vi "Main.vi"(11 "Module Admin":refnum<class "Delacor_lib_QMH_Module Admin.lvclass">) -> ()   [LabVIEW 2019, in "Spectrometer.lvlib"]
doc: "This template is based off of the Queued Message Handler design pattern and the Queued Message Handler project template that ships with LabVIEW.\n\nThe main difference is that the queue is private to this module and communication between modules is performed via Broadcast and Request events.\n\nRequest events are wrapped in public API methods and are handled in the Event Handling Loop (EHL) of this VI. Any module can register for Broadcast events sent by this module. The EHL generates messages based on user interface actions.\n\nThe Message Handling Loop (MHL) processes messages generated by the EHL, or by other messages. The messages are string values, so new messages can be added easily to the Message Cases case structure in the MHL. Each message cluster can also provide an optional value for Message Data, which is a variant that can be converted to whatever message-specific data is required.\n_____\nBased on Delacor QMH Project Template 5.0.0.82."
uses:
  Spectrometer.lvlib
  <vilib>/Delacor/Delacor QMH/Libraries/Module Admin_class/Delacor_lib_QMH_Module Admin.lvclass
  Module Data--cluster.ctl
  Spectrometer-LVClass/Abstract Spectrometer_class/Abstract Spectrometer.lvclass
  <vilib>/Delacor/Delacor QMH/Libraries/Message Queue_class/Delacor_lib_QMH_Message Queue.lvclass/Delacor_lib_QMH_Message Queue.ctl
  Stop Argument--cluster.ctl
  <vilib>/Delacor/Delacor QMH/Libraries/Module Admin_class/Delacor_lib_QMH_Module Admin.lvclass/Delacor_lib_QMH_Module Admin.ctl
  Set Wavelength Argument--cluster.ctl
  Set Wavelength (Reply Payload)--cluster.ctl
  Set Slit Width Argument--cluster.ctl
  Set Slit Width (Reply Payload)--cluster.ctl
  Set Grating Argument--cluster.ctl
  Set Grating (Reply Payload)--cluster.ctl
  Get Module Data Argument--cluster.ctl
  Get Module Data (Reply Payload)--cluster.ctl
  <vilib>/Utility/miscctls.llb/LVPointTypeDef.ctl
  Spectrometer-LVClass/Simulated_class/Simulated.lvclass
  C:/Users/Michael/Documents/GitHub/CampenLab/Spectrometer-LVClass/Abstract Spectrometer_class/Abstract Spectrometer.lvclass
  <vilib>/Delacor/Delacor QMH/Libraries/Message Queue_class/Delacor_lib_QMH_Enqueue Message (Single).vi
  <vilib>/Delacor/Delacor QMH/Libraries/Module Admin_class/Delacor_lib_QMH_Get External Launch.vi
  <vilib>/Utility/error.llb/Error Cluster From Error Code.vi
  <vilib>/ErrorRing/Error Ring.xnode
  <vilib>/Delacor/Delacor QMH/Libraries/Message Queue_class/Delacor_lib_QMH_Message Queue.lvclass
panel:
  in  "Spectrometer Class":u16(ring) items=["Simulated", "SpectraPro HRS"]
  out "Status":string
  in  "Simulate MHL Error":bool
  in  "Simulate EHL Error":bool
  out "error out":errorcluster
  # "SpectraPro"
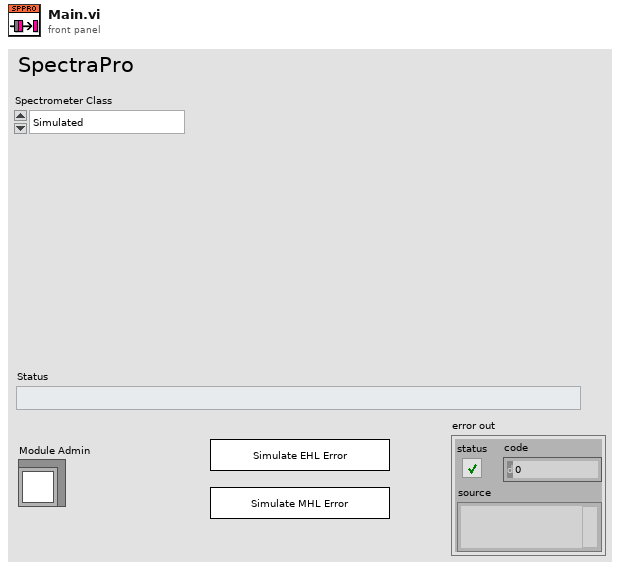
[diagram p1: front panel]
types:
  T1 = typedef "Spectrometer.lvlib/Request Events--cluster.ctl" = cluster{"Stop Module":refnum<user-event>, "Show Panel":refnum<user-event>, "Hide Panel":refnum<user-event>, "Get Module Execution Status":refnum<user-event>, "Show Diagram":refnum<user-event>, "Set Wavelength":refnum<user-event>, "Set Slit Width":refnum<user-event>, "Set Grating":refnum<user-event>, "Get Module Data":refnum<user-event>}
  T2 = typedef "Spectrometer.lvlib/Module Data--cluster.ctl" = cluster{"Status":string, "-Abstract Spectrometer.lvclass":refnum<class "Abstract Spectrometer.lvclass">, "Device Data":cluster{"Wavelength":dbl, "Slit Width":dbl, "Grating ID":u32}}
  T3 = enum32{"invalid lock state", "Not Locked", "Locked (No Password)", "Password-protected"}
  T4 = typedef "Spectrometer.lvlib/Stop Argument--cluster.ctl" = cluster{"Origin":string, "Exit via Stop Module Req?":bool, "Wait for Module to stop?":bool}
  T5 = typedef "Spectrometer.lvlib/Set Wavelength Argument--cluster.ctl" = cluster{"Wavelength":dbl, "Wait Notifier":refnum<notifier>, "wait for reply":bool}
  T6 = typedef "Spectrometer.lvlib/Set Slit Width Argument--cluster.ctl" = cluster{"Slit Width (um)":dbl, "Wait Notifier":refnum<notifier>, "wait for reply":bool}
  T7 = typedef "Spectrometer.lvlib/Set Grating Argument--cluster.ctl" = cluster{"Grating ID":u32, "Wait Notifier":refnum<notifier>, "wait for reply":bool}
  T8 = typedef "Spectrometer.lvlib/Get Module Data Argument--cluster.ctl" = cluster{"Wait Notifier":refnum<notifier>, "wait for reply":bool}
  T9 = typedef "LVPointTypeDef.ctl" = cluster{"Horizontal":i16, "Vertical":i16}
  T10 = enum32{"Invalid", "Standard", "Closed", "Hidden", "Minimized", "Maximized"}
  T11 = typedef "Spectrometer.lvlib/Set Wavelength (Reply Payload)--cluster.ctl" = cluster{"Wavelength":dbl, "Set Wavelength_error":errorcluster}
  T12 = typedef "Spectrometer.lvlib/Set Slit Width (Reply Payload)--cluster.ctl" = cluster{"Slit Width (um)":dbl, "Set Slit Width_error":errorcluster}
  T13 = typedef "Spectrometer.lvlib/Set Grating (Reply Payload)--cluster.ctl" = cluster{"Grating ID":u32, "Set Grating_error":errorcluster}
  T14 = typedef "Spectrometer.lvlib/Get Module Data (Reply Payload)--cluster.ctl" = cluster{"Spectrometer":T2, "Get Module Data_error":errorcluster}
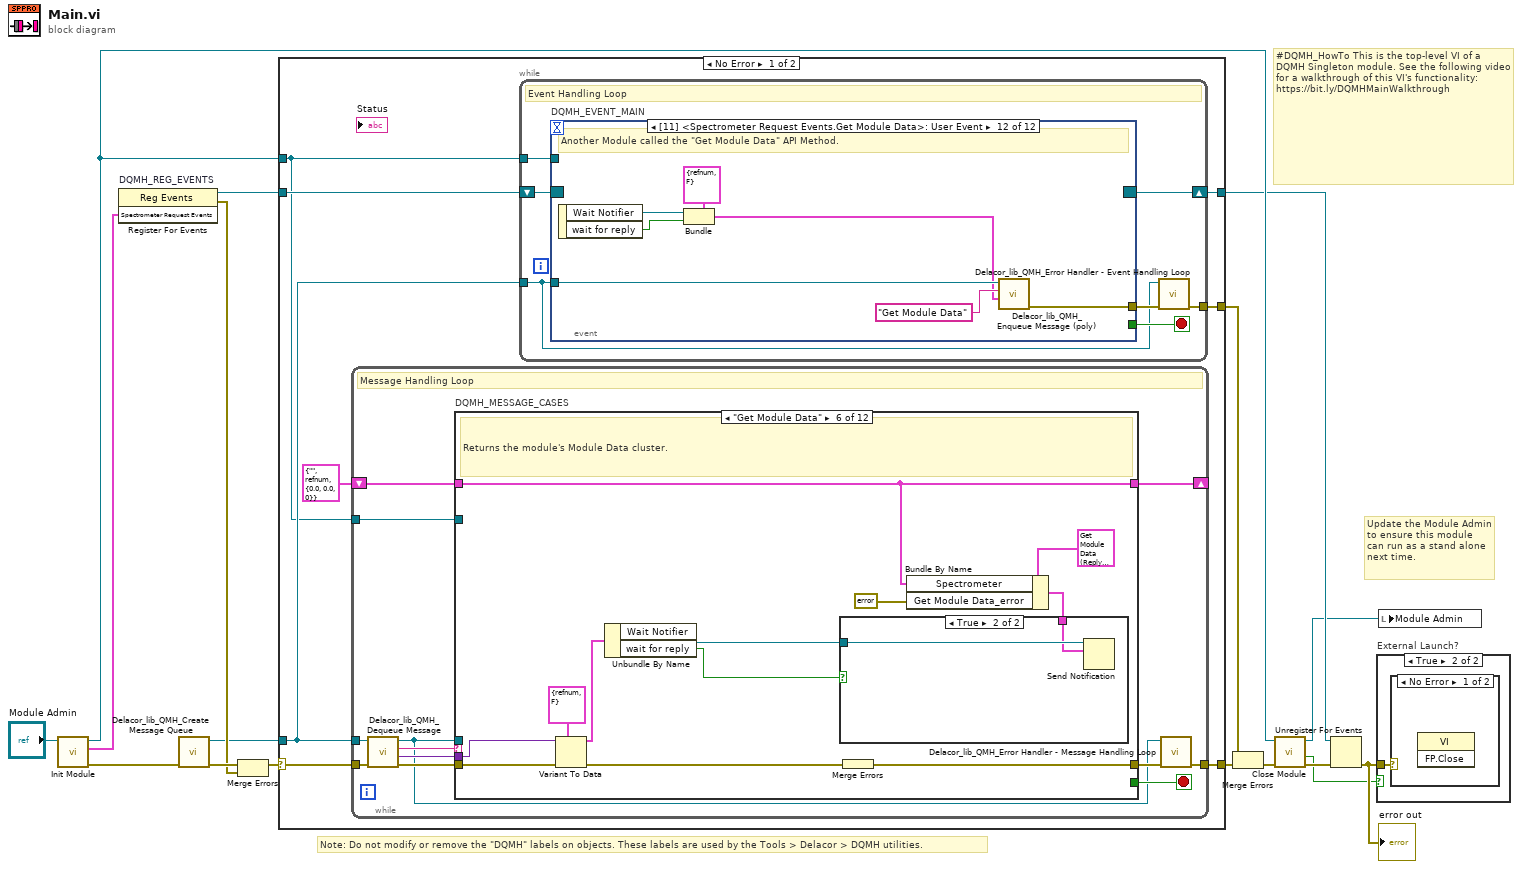
[diagram p0: block diagram]
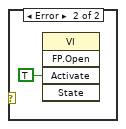
[diagram p3: hidden frame]
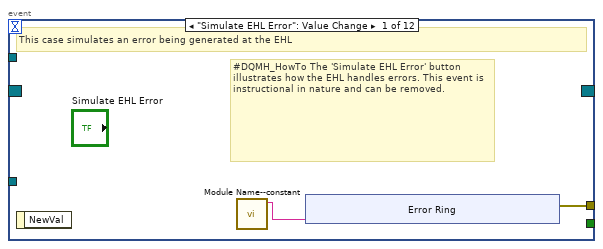
[diagram p4: hidden frame]
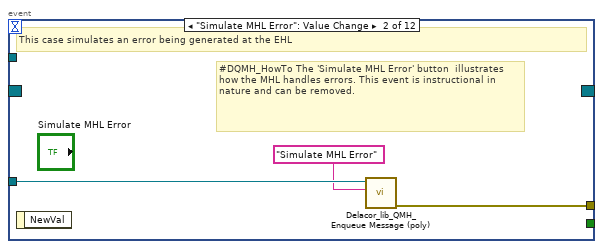
[diagram p5: hidden frame]
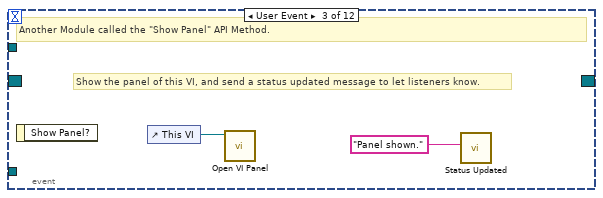
[diagram p6: hidden frame]
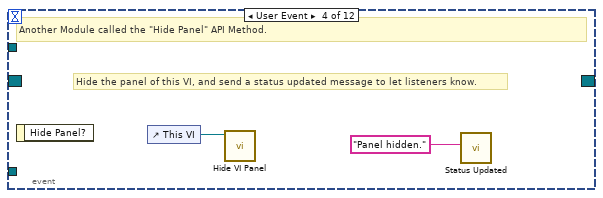
[diagram p7: hidden frame]
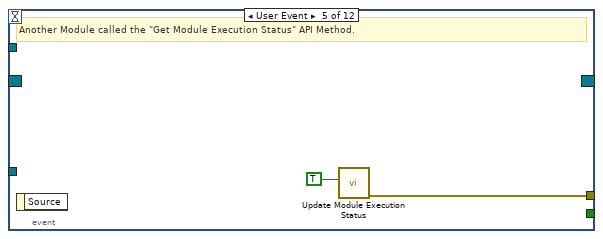
[diagram p8: hidden frame]
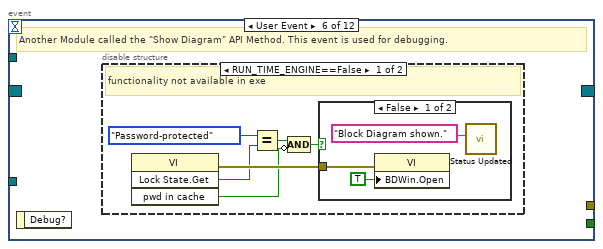
[diagram p9: hidden frame]
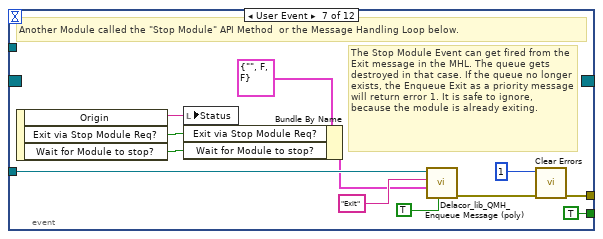
[diagram p12: hidden frame]
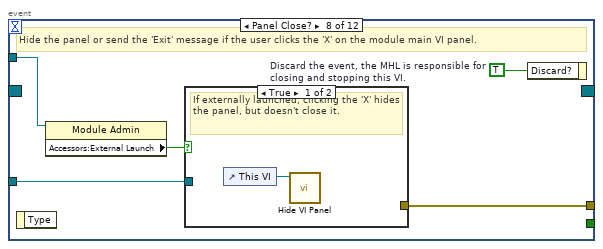
[diagram p13: hidden frame]
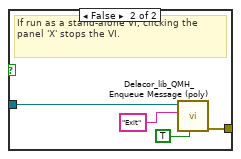
[diagram p14: hidden frame]
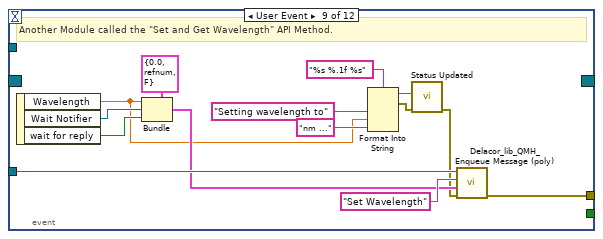
[diagram p15: hidden frame]
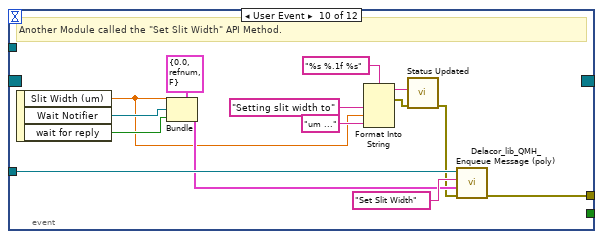
[diagram p16: hidden frame]
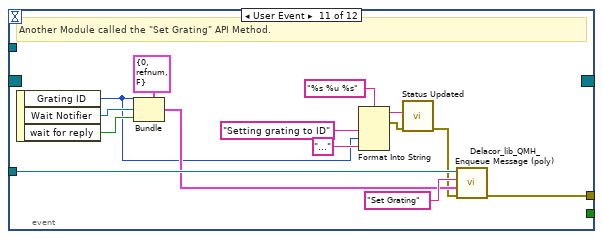
[diagram p17: hidden frame]
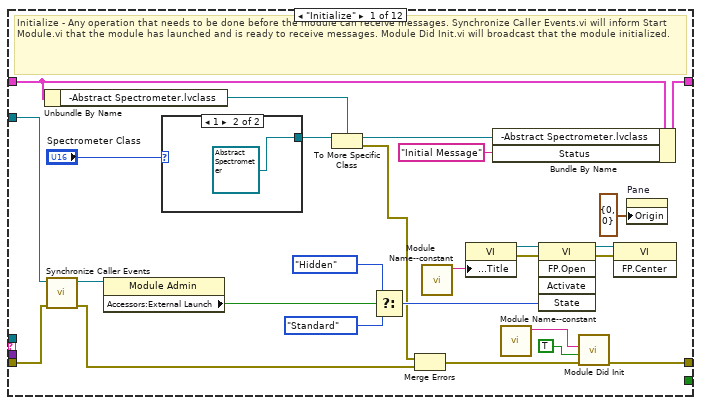
[diagram p18: hidden frame]
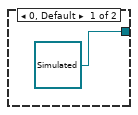
[diagram p19: hidden frame]
diagram:
  # "#DQMH_HowTo This is the top-level VI of a DQMH Singleton module. See the following video for a walkthrough of this VI's functionality: https://bit.ly/DQMHMainWalkthrough"
  # "Note: Do not modify or remove the \"DQMH\" labels on objects. These labels are used by the Tools > Delacor > DQMH utilities."
  # "Update the Module Admin to ensure this module can run as a stand alone next time."
  n1 = call "Init Module.vi"("Singleton Module Admin in"="Module Admin") -> ("error out"=w16:errorcluster, "Spectrometer Request Events"=w5:T1, "Singleton Module Admin out"=w8:refnum<class "Delacor_lib_QMH_Module Admin.lvclass">)  [unwired: 8 in]
  n2 = register-events "DQMH_REG_EVENTS"(w5) -> (reference out=w6:refnum<event-registration>, error out=w9:errorcluster)  [unwired: 2 in]
  n3 = call <vilib>:"Delacor_lib_QMH_Create Message Queue.vi"("error in (no error)"=w16) -> ("error out"=w11:errorcluster, "Message Queue"=w4:refnum<class "Delacor_lib_QMH_Message Queue.lvclass">)  [unwired: 9 in]
  n4 = Merge Errors(w11, w9) -> (w10:errorcluster)
  n5 = case shown="No Error" w10 {
    selector: w10 -> [w23 w326]
    tunnel: [w25 w325] -> w17
    tunnel: [w22 w331] -> w7
    tunnel: w6 -> [w20 w331]
    tunnel: w4 -> [w19 w324]
    tunnel: [w24 _] -> w14
    tunnel: w8 -> [w18 w327]
    frame No Error {
      n6 = while {
        tunnel: w19 -> [w133]
        shift-right: [w137] -> _
        shift-left: T2 {"Status"="", "-Abstract Spectrometer.lvclass"=refnum, "Device Data"={"Wavelength"=0.0, "Slit Width"=0.0, "Grating ID"=0}} ("Data Cluster") -> [w138]
        tunnel: w23 -> [w141]
        tunnel: [w139] -> w25
        tunnel: w18 -> [w131]
        stop <- w136 stop-if-true
        # "Message Handling Loop"
        n7 = call-dynamic "Delacor_lib_QMH_Dequeue Message.vi"("error in (no error)"=w141, "Message Queue in"=w133) -> ("error out"=w140:errorcluster, "Message Data"=w134:variant, "Message"=w135:string, "Message Queue out"=w132:refnum<class "Delacor_lib_QMH_Message Queue.lvclass">)  [unwired: 6 in]
        n8 = case "DQMH_MESSAGE_CASES" shown="\"Get Module Data\"" w135 {
          selector: w135 -> [_ _ _ _ _ _ _ _ _ _ _ w311]
          tunnel: w132 -> [_ _ _ _ _ _ _ _ _ w281 w303 _]
          tunnel: w140 -> [w166 w172 w189 w214 w239 w258 w263 w265 w270 w288 w309 w313]
          tunnel: [w164 w172 w182 w206 w231 w249 w262 w265 w269 w284 w306 w314] -> w142
          tunnel: w138 -> [w147 w171 w180 w205 w230 w248 w261 w264 w267 w283 w302 w312]
          tunnel: [w155 w171 w181 w203 w229 w248 w261 w264 w267 w283 w302 w312] -> w137
          tunnel: [_ _ _ _ _ _ _ _ _ _ w301 _] -> w136
          tunnel: w134 -> [_ _ w188 w212 w237 w256 _ _ _ w282 w300 _]
          tunnel: w131 -> [w156 _ _ _ _ _ _ _ _ w280 w295 _]
          frame "Initialize" {
            # "Initialize - Any operation that needs to be done before the module can receive messages. Synchronize Caller Events.vi will inform Start Module.vi that the module has launched and is ready to receive messages. Module Did Init.vi will broadcast that the module initialized."
            n9 = Unbundle By Name(w147) -> ("-Abstract Spectrometer.lvclass"=w146:refnum<class "Abstract Spectrometer.lvclass">)
            n10 = call "Synchronize Caller Events.vi"("error in (no error)"=w166, "Singleton Module Admin in"=w156) -> ("error out"=w165:errorcluster, "Singleton Module Admin out"=w152:refnum<class "Delacor_lib_QMH_Module Admin.lvclass">)  [unwired: 8 in]
            n11 = property class="Module Admin"(reference=w152) -> ("Accessors:External Launch"=w160:bool)  [unwired: 1 in, 2 out]
            n12 = case shown="1" "Spectrometer Class" {
              tunnel: [refnum<class "Simulated.lvclass"> refnum ("Simulated") refnum<class "Abstract Spectrometer.lvclass"> refnum ("Abstract Spectrometer.lvclass")] -> w143
              frame 0, Default {
              }
              frame 1 {
              }
            }
            n13 = To More Specific Class(target class=w146, reference=w143) -> (specific class reference=w148:refnum<class "Abstract Spectrometer.lvclass">, error out=w145:errorcluster)  [unwired: 1 in]
            n14 = Select(t=T10."Hidden" ("State"), s=w160, f=T10."Standard" ("State")) -> (s? t:f=w157:T10)
            n15 = Merge Errors(w145, w165) -> (w150:errorcluster)
            n16 = call "Module Name--constant.vi"() -> ("Module Name"=w163:string)  [unwired: 11 in]
            n17 = property class="VI"("Front Panel.Title"=w163) -> (reference out=w162:refnum<vi>, error out=w168:errorcluster)  [unwired: 2 in]
            n18 = Bundle By Name(cluster=w147, "-Abstract Spectrometer.lvclass"=w148, "Status"="Initial Message") -> (w155:T2)
            n19 = call "Module Name--constant.vi"() -> ("Module Name"=w153:string)  [unwired: 11 in]
            n20 = invoke class="VI" method="FP.Open"(reference=w162, error in=w168, "State"=w157) -> (reference out=w161:refnum<vi>, error out=w167:errorcluster)  [unwired: 2 in, 3 out]
            n21 = call "Module Did Init.vi"("error in (no error)"=w150, "Initialized?"=TRUE, "Origin"=w153) -> ("error out"=w164:errorcluster)  [unwired: 8 in]
            n22 = invoke class="VI" method="FP.Center"(reference=w161, error in=w167) -> ()  [unwired: 1 in, 3 out]
            n23 = property on="Pane" class="Pane"("Origin"=T9 {"Horizontal"=0, "Vertical"=0}) -> ()  [unwired: 2 in, 2 out]
          }
          frame "--- Module Specific ---" {
            # "Separator -- The following cases handle messages specific to this Module."
          }
          frame "Set Wavelength" {
            # "#TODO: Update status when\nwavelength is set."
            # "Set the wavelength (nm). After setting the wavelength we confirm that the spectrometer is set to the desired wavelength."
            n24 = Unbundle By Name(w180) -> ("-Abstract Spectrometer.lvclass"=w179:refnum<class "Abstract Spectrometer.lvclass">)
            n25 = Variant To Data(error in=w189, type=T5 {"Wavelength"=0.0, "Wait Notifier"=refnum, "wait for reply"=FALSE} ("Set and Get Wavelength Argument"), Variant=w188) -> (data=w186:T5, error out=w175:errorcluster)
            n26 = Unbundle By Name(w186) -> ("Wavelength"=w174:dbl, "Wait Notifier"=w185:refnum<notifier>, "wait for reply"=w176:bool)
            n27 = call-dynamic "Set Wavelength.vi"("Wait for Reply"=w176, "Wavelength (nm)"=w174, "Abstract Spectrometer in"=w179) -> ("error out"=w178:errorcluster, "Wavelength (nm) out"=w173:dbl, "Abstract Spectrometer out"=w177:refnum<class "Abstract Spectrometer.lvclass">)  [unwired: 6 in]
            n28 = Merge Errors(w178, w175) -> (w182:errorcluster)
            n29 = Bundle By Name(cluster=w180, "Device Data.Wavelength"=w173, "-Abstract Spectrometer.lvclass"=w177) -> (w181:T2)
            n30 = Bundle By Name(cluster=T11 {"Wavelength"=0.0, "Set Wavelength_error"={"status"=FALSE, "code"=0, "source"=""}} ("Set and Get Wavelength (Reply Payload)"), "Wavelength"=w173, "Set Wavelength_error"=w178) -> (w184:T11)
            n31 = case shown="True" w176 {
              tunnel: w185 -> [_ w197]
              tunnel: w184 -> [_ w196]
              tunnel: w173 -> [_ w190]
              frame False {
              }
              frame True {
                n32 = Format Into String(format string="%s %.1f %s", "Wavelength set to " ("input 1"), w190, "nm" ("input 3")) -> (resulting string=w193:string, error out=w194:errorcluster)  [unwired: 2 in]
                n33 = call "Status Updated.vi"("error in (no error)"=w194, "Status"=w193) -> ()  [unwired: 9 in, 1 out]
                n34 = Send Notification(notification=w196, notifier=w197) -> ()  [unwired: 1 in, 2 out]
              }
            }
            n35 = call "Broadcast Wavelength.vi"("Reply Payload"=w184) -> ()  [unwired: 10 in, 1 out]
          }
          frame "Set Slit Width" {
            # "Sets the slit width of the spectrometer. If 'Wait for Reply' is true, VI executes util the slit width is set."
            n36 = Unbundle By Name(w205) -> ("-Abstract Spectrometer.lvclass"=w204:refnum<class "Abstract Spectrometer.lvclass">)
            n37 = Variant To Data(error in=w214, type=T6 {"Slit Width (um)"=0.0, "Wait Notifier"=refnum, "wait for reply"=FALSE} ("Set Slit Width Argument"), Variant=w212) -> (data=w210:T6, error out=w213:errorcluster)
            n38 = Unbundle By Name(w210) -> ("Slit Width (um)"=w200:dbl, "wait for reply"=w201:bool, "Wait Notifier"=w209:refnum<notifier>)
            n39 = call-dynamic "Set Slit Width.vi"("Wait for Reply"=w201, "Slit Width (um)"=w200, "Abstract Spectrometer in"=w204) -> ("error out"=w199:errorcluster, "Slit Width (um) out"=w198:dbl, "Abstract Spectrometer out"=w202:refnum<class "Abstract Spectrometer.lvclass">)  [unwired: 6 in]
            n40 = Bundle By Name(cluster=w205, "-Abstract Spectrometer.lvclass"=w202, "Device Data.Slit Width"=w198) -> (w203:T2)
            n41 = Merge Errors(w213, w199) -> (w206:errorcluster)
            n42 = Bundle By Name(cluster=T12 {"Slit Width (um)"=0.0, "Set Slit Width_error"={"status"=FALSE, "code"=0, "source"=""}} ("Set Slit Width (Reply Payload)"), "Slit Width (um)"=w198, "Set Slit Width_error"=w199) -> (w208:T12)
            n43 = case shown="True" w201 {
              tunnel: w209 -> [_ w222]
              tunnel: w208 -> [_ w221]
              tunnel: w198 -> [_ w215]
              frame False {
              }
              frame True {
                n44 = Format Into String(format string="%s %.1f %s", "Slit width set to " ("input 1"), w215, "um" ("input 3")) -> (resulting string=w218:string, error out=w219:errorcluster)  [unwired: 2 in]
                n45 = call "Status Updated.vi"("error in (no error)"=w219, "Status"=w218) -> ()  [unwired: 9 in, 1 out]
                n46 = Send Notification(notification=w221, notifier=w222) -> ()  [unwired: 1 in, 2 out]
              }
            }
            n47 = call "Broadcast Slit Width.vi"("Reply Payload"=w208) -> ()  [unwired: 10 in, 1 out]
          }
          frame "Set Grating" {
            # "Switch to the grating with the specified ID. The grating ID is then broadcasted."
            n48 = Variant To Data(error in=w239, type=T7 {"Grating ID"=0, "Wait Notifier"=refnum, "wait for reply"=FALSE} ("Set Grating Argument"), Variant=w237) -> (data=w235:T7, error out=w238:errorcluster)
            n49 = Unbundle By Name(w230) -> ("-Abstract Spectrometer.lvclass"=w228:refnum<class "Abstract Spectrometer.lvclass">)
            n50 = Unbundle By Name(w235) -> ("Grating ID"=w225:u32, "Wait Notifier"=w234:refnum<notifier>, "wait for reply"=w226:bool)
            n51 = call-dynamic "Set Grating.vi"("Wait for Reply?"=w226, "Grating ID"=w225, "Abstract Spectrometer in"=w228) -> ("error out"=w224:errorcluster, "Grating ID out"=w223:u32, "Abstract Spectrometer out"=w227:refnum<class "Abstract Spectrometer.lvclass">)  [unwired: 6 in]
            n52 = Merge Errors(w238, w224) -> (w231:errorcluster)
            n53 = Bundle By Name(cluster=T13 {"Grating ID"=0, "Set Grating_error"={"status"=FALSE, "code"=0, "source"=""}} ("Set Grating (Reply Payload)"), "Grating ID"=w223, "Set Grating_error"=w224) -> (w233:T13)
            n54 = case shown="True" w226 {
              tunnel: w234 -> [_ w246]
              tunnel: w233 -> [_ w245]
              tunnel: w223 -> [_ w240]
              frame False {
              }
              frame True {
                n55 = Format Into String(format string="%s %u", "Grating set to ID" ("input 1"), w240) -> (resulting string=w243:string, error out=w244:errorcluster)  [unwired: 2 in]
                n56 = call "Status Updated.vi"("error in (no error)"=w244, "Status"=w243) -> ()  [unwired: 9 in, 1 out]
                n57 = Send Notification(notification=w245, notifier=w246) -> ()  [unwired: 1 in, 2 out]
              }
            }
            n58 = Bundle By Name(cluster=w230, "-Abstract Spectrometer.lvclass"=w227, "Device Data.Grating ID"=w223) -> (w229:T2)
            n59 = call "Broadcast Grating.vi"("Reply Payload"=w233) -> ()  [unwired: 10 in, 1 out]
          }
          frame "Get Module Data" {
            # "Returns the module's Module Data cluster."
            n60 = Variant To Data(error in=w258, type=T8 {"Wait Notifier"=refnum, "wait for reply"=FALSE} ("Get Module Data Argument"), Variant=w256) -> (data=w254:T8, error out=w257:errorcluster)
            n61 = Unbundle By Name(w254) -> ("Wait Notifier"=w253:refnum<notifier>, "wait for reply"=w252:bool)
            n62 = Merge Errors(w257) -> (w249:errorcluster)
            n63 = Bundle By Name(cluster=T14 {"Spectrometer"={"Status"="", "-Abstract Spectrometer.lvclass"=refnum, "Device Data"={"Wavelength"=0.0, "Slit Width"=0.0, "Grating ID"=0}}, "Get Module Data_error"={"status"=FALSE, "code"=0, "source"=""}} ("Get Module Data (Reply Payload)"), "Spectrometer"=w248, "Get Module Data_error"=errorcluster {"status"=FALSE, "code"=0, "source"=""}) -> (w251:T14)
            n64 = case shown="True" w252 {
              tunnel: w253 -> [_ w260]
              tunnel: w251 -> [_ w259]
              frame False {
              }
              frame True {
                n65 = Send Notification(notification=w259, notifier=w260) -> ()  [unwired: 1 in, 2 out]
              }
            }
          }
          frame "---Copy This Frame---" {
            # "Duplicate this frame when creating new messages.  Change this comment in the duplicated frame to describe this message."
            n66 = Merge Errors(w263) -> (w262:errorcluster)
          }
          frame "--- Exit and Error Handling---" {
            # "Separator - The following cases handle errors and exit messages."
          }
          frame "Simulate MHL Error" {
            # "#DQMH_HowTo The 'Simulate MHL Error' button  illustrates how the MHL handles errors. This event is instructional in nature and can be removed."
            # "Simulate an error occurring at the MHL"
            n67 = call "Module Name--constant.vi"() -> ("Module Name"=w266:string)  [unwired: 11 in]
            n68 = xnode "Error Ring"("parameter 0"=w266) -> ("error out"=w268:errorcluster)
            n69 = Merge Errors(w270, w268) -> (w269:errorcluster)
          }
          frame "Error" {
            # "#CodeRecommended - If you ever change the name of this \"Error\" message, you'll need to update the name in the Check Loop Error.vi as well."
            # "#CodeRecommended - If the module is running in standalone mode (External Launch = FALSE), this code will pop up an error dialog and call the 'Exit' message if an error occurs. Add more fine-grained error handling here."
            # "Error - Check the error message data and respond accordingly. This message is sent by the \"Error Handler\" VIs at the end of each loop in this application."
            n70 = property class="Module Admin"(reference=w280) -> ("Accessors:External Launch"=w279:bool)  [unwired: 1 in, 2 out]
            n71 = Variant To Data(error in=w288, type=errorcluster {"status"=FALSE, "code"=0, "source"=""} ("error constant"), Variant=w282) -> (data=w289:errorcluster, error out=w286:errorcluster)
            n72 = call "Module Name--constant.vi"() -> ("Module Name"=w278:string)  [unwired: 11 in]
            n73 = call "Error Reported.vi"("Additional Information"=w278, "Error"=w289) -> ()  [unwired: 9 in, 1 out]
            n74 = case shown="False" w279 {
              tunnel: [w294 _] -> w285
              tunnel: w281 -> [w292 _]
              tunnel: w289 -> [w293 _]
              frame False {
                # "If the module is running standalone, then pop up an error dialog and call the \"Exit\" message."
                n75 = call <vilib>:"Simple Error Handler.vi"("error in (no error)"=w293) -> ()  [unwired: 4 in, 5 out]
                n76 = call-poly <vilib>:"Delacor_lib_QMH_Enqueue Message (poly).vi"("Priority Message? (F)"=TRUE, "Message"="Exit", "Message Queue in"=w292) -> ("error out"=w294:errorcluster)  [unwired: 7 in, 1 out]
              }
              frame True {
                # "If the module was launched externally, calling the Error Reported broadcast VI is the only action performed by the \"Error\" message. The module's caller can then process the error appropriately."
              }
            }
            n77 = Merge Errors(w286, w285) -> (w284:errorcluster)
            n78 = local write "error out"(w284) -> ()
          }
          frame "Exit" {
            w299 = 91  # 91: not all Exit messages will have an argument
            w301 = TRUE  # Stop the VI
            # "Release the message queue reference"
            # "#CodeNeeded - Add any required cleanup code here"
            # "Exit - Exit the application."
            n79 = Variant To Data(error in=w309, type=T4 {"Origin"="", "Exit via Stop Module Req?"=FALSE, "Wait for Module to stop?"=FALSE} ("Stop Argument"), Variant=w300) -> (data=w297:T4, error out=w305:errorcluster)
            n80 = call <vilib>:"Clear Errors.vi"("error in (no error)"=w305, "specific error code to clear (0: all)"=w299) -> ("error out"=w308:errorcluster)  [unwired: 4 in, 1 out]
            n81 = control-ref of="This VI"() -> (w296:refnum<vi>)
            n82 = call-dynamic "Delacor_lib_QMH_Release Message Queue.vi"("error in (no error)"=w308, "Message Queue"=w303) -> ("error out"=w307:errorcluster)  [unwired: 9 in]
            n83 = call "Handle Exit.vi"("Stop Argument"=w297, "Admin in"=w295, "VI reference"=w296) -> ("error out"=w304:errorcluster)  [unwired: 7 in, 1 out]
            n84 = Merge Errors(w307, w304) -> (w306:errorcluster)
          }
          frame Default {
            # "'Default' case only runs if there is a message that isn't defined in any of the other cases.  Output a programming error."
            n85 = call "Module Name--constant.vi"() -> ("Module Name"=w310:string)  [unwired: 11 in]
            n86 = xnode "Error Ring"("parameter 0"=w311, "parameter 1"=w310) -> ("error out"=w315:errorcluster)
            n87 = Merge Errors(w313, w315) -> (w314:errorcluster)
          }
        }
        n88 = call-dynamic "Delacor_lib_QMH_Error Handler - Message Handling Loop.vi"("error in (no error)"=w142, "Message Queue in"=w132) -> ("dup error in"=w139:errorcluster)  [unwired: 8 in, 1 out]
      }
      n89 = while {
        tunnel: w19 -> [w26]
        shift-right: [w29] -> w22
        shift-left: w20 -> [w30]
        tunnel: [w31] -> w24
        tunnel: w18 -> [w27]
        stop <- w28 stop-if-true
        # "Event Handling Loop"
        n90 = event "DQMH_EVENT_MAIN" shown="[11] <Spectrometer Request Events.Get Module Data>: User Event" {
          selector: w30 -> [_ _ _ _ _ _ _ _ _ _ _ _]
          dyn-events: [_ _ _ _ _ _ _ _ _ _ _ _] -> w29
          timeout: _ -> [_ _ _ _ _ _ _ _ _ _ _ _]
          tunnel: [_ _ _ _ _ _ TRUE ("Discard?") _ _ _ _ _] -> w28
          tunnel: w26 -> [_ w43 _ _ _ _ w67 w74 w95 w109 w123 w130]
          tunnel: [w34 w44 _ _ w50 _ w70 w76 w89 w105 w117 w124] -> w32
          tunnel: w27 -> [_ _ _ _ _ _ _ w73 _ _ _ _]
          event "Simulate EHL Error": Value Change {
            # "#DQMH_HowTo The 'Simulate EHL Error' button  illustrates how the EHL handles errors. This event is instructional in nature and can be removed."
            # "This case simulates an error being generated at the EHL"
            n91 = event-data() -> ()  [unwired: 1 in, 1 out]
            n92 = call "Module Name--constant.vi"() -> ("Module Name"=w33:string)  [unwired: 11 in]
            n93 = xnode "Error Ring"("parameter 0"=w33) -> ("error out"=w34:errorcluster)
          }
          event "Simulate MHL Error": Value Change {
            # "#DQMH_HowTo The 'Simulate MHL Error' button  illustrates how the MHL handles errors. This event is instructional in nature and can be removed."
            # "This case simulates an error being generated at the EHL"
            n94 = event-data() -> ()  [unwired: 1 in, 1 out]
            n95 = call-poly <vilib>:"Delacor_lib_QMH_Enqueue Message (poly).vi"("Message"="Simulate MHL Error", "Message Queue in"=w43) -> ("error out"=w44:errorcluster)  [unwired: 8 in, 1 out]
          }
          event User Event {
            # "Show the panel of this VI, and send a status updated message to let listeners know."
            # "Another Module called the \"Show Panel\" API Method."
            n96 = event-data() -> ()  [unwired: 1 in, 1 out]
            n97 = control-ref of="This VI"() -> (w46:refnum<vi>)
            n98 = call "Open VI Panel.vi"("VI"=w46) -> ()  [unwired: 10 in, 1 out]
            n99 = call "Status Updated.vi"("Status"="Panel shown." ("format string")) -> ()  [unwired: 10 in, 1 out]
          }
          event User Event {
            # "Hide the panel of this VI, and send a status updated message to let listeners know."
            # "Another Module called the \"Hide Panel\" API Method."
            n100 = event-data() -> ()  [unwired: 1 in, 1 out]
            n101 = control-ref of="This VI"() -> (w48:refnum<vi>)
            n102 = call "Hide VI Panel.vi"("VI"=w48) -> ()  [unwired: 10 in, 1 out]
            n103 = call "Status Updated.vi"("Status"="Panel hidden." ("format string")) -> ()  [unwired: 10 in, 1 out]
          }
          event User Event {
            # "Another Module called the \"Get Module Execution Status\" API Method."
            n104 = event-data() -> ()  [unwired: 1 in, 1 out]
            n105 = call "Update Module Execution Status.vi"("Running?"=TRUE) -> ("error out"=w50:errorcluster)  [unwired: 10 in]
          }
          event User Event {
            # "Another Module called the \"Show Diagram\" API Method. This event is used for debugging."
            n106 = event-data() -> ()  [unwired: 1 in, 1 out]
            n107 = disable-structure shown="RUN_TIME_ENGINE==False" {
              frame condition #0 (active) {
                # "functionality not available in exe"
                n108 = invoke class="VI" method="Lock State.Get"() -> (error out=w56:errorcluster, "Get Lock State"=w55:T3, "pwd in cache"=w52:bool)  [unwired: 4 in, 1 out]
                n109 = Equal?(x=T3."Password-protected", y=w55) -> (x = y?=w53:bool)
                n110 = Compound Arithmetic op=AND(w53, invert w52) -> (w51:bool)
                n111 = case shown="False" w51 {
                  tunnel: w56 -> [w59 _]
                  frame False {
                    n112 = property class="VI"(error in=w59, "BDWin.Open"=TRUE ("Block Diagram Window:Open")) -> ()  [unwired: 1 in, 2 out]
                    n113 = call "Status Updated.vi"("Status"="Block Diagram shown." ("format string")) -> ()  [unwired: 10 in, 1 out]
                  }
                  frame True {
                    # "Password-protected VI, and the password is not in the cache. Do not show the diagram."
                  }
                }
              }
              frame condition #1 {
              }
            }
          }
          event User Event {
            # "The Stop Module Event can get fired from the Exit message in the MHL. The queue gets destroyed in that case. If the queue no longer exists, the Enqueue Exit as a priority message will return error 1. It is safe to ignore, because the module is already exiting."
            # "Another Module called the \"Stop Module\" API Method  or the Message Handling Loop below."
            n114 = event-data() -> ("Origin"=w66:string, "Exit via Stop Module Req?"=w62:bool, "Wait for Module to stop?"=w61:bool)  [unwired: 1 in]
            n115 = local write "Status"(w66) -> ()
            n116 = Bundle By Name(cluster=T4 {"Origin"="", "Exit via Stop Module Req?"=FALSE, "Wait for Module to stop?"=FALSE} ("Stop Argument"), "Exit via Stop Module Req?"=w62, "Wait for Module to stop?"=w61) -> (w60:T4)
            n117 = call-poly <vilib>:"Delacor_lib_QMH_Enqueue Message (poly).vi"("Priority Message? (F)"=TRUE, "Message Data"=w60, "Message"="Exit", "Message Queue in"=w67) -> ("error out"=w71:errorcluster)  [unwired: 6 in, 1 out]
            n118 = call <vilib>:"Clear Errors.vi"("error in (no error)"=w71, "specific error code to clear (0: all)"=1) -> ("error out"=w70:errorcluster)  [unwired: 4 in, 1 out]
          }
          event Panel Close? {
            w75 = TRUE  # Discard the event, the MHL is responsible for closing and stopping this VI.
            # "Hide the panel or send the 'Exit' message if the user clicks the 'X' on the module main VI panel."
            n119 = event-data() -> ()  [unwired: 1 in, 1 out]
            n120 = property class="Module Admin"(reference=w73) -> ("Accessors:External Launch"=w72:bool)  [unwired: 1 in, 2 out]
            n121 = case shown="True" w72 {
              tunnel: w74 -> [_ w80]
              tunnel: [_ w81] -> w76
              frame True {
                # "If externally launched, clicking the 'X' hides the panel, but doesn't close it."
                n122 = control-ref of="This VI"() -> (w77:refnum<vi>)
                n123 = call "Hide VI Panel.vi"("VI"=w77) -> ()  [unwired: 10 in, 1 out]
              }
              frame False {
                # "If run as a stand-alone VI, clicking the panel 'X' stops the VI."
                n124 = call-poly <vilib>:"Delacor_lib_QMH_Enqueue Message (poly).vi"("Priority Message? (F)"=TRUE, "Message"="Exit", "Message Queue in"=w80) -> ("error out"=w81:errorcluster)  [unwired: 7 in, 1 out]
              }
            }
            n125 = event-data("Discard?"=w75) -> ()  [unwired: 1 in, 1 out]
          }
          event User Event {
            # "Another Module called the \"Set and Get Wavelength\" API Method."
            n126 = event-data() -> ("Wavelength"=w83:dbl, "Wait Notifier"=w91:refnum<notifier>, "wait for reply"=w90:bool)  [unwired: 1 in]
            n127 = Bundle(cluster=T5 {"Wavelength"=0.0, "Wait Notifier"=refnum, "wait for reply"=FALSE} ("Set and Get Wavelength Argument"), "Wavelength"=w83, "Wait Notifier"=w91, "wait for reply"=w90) -> (w92:T5)
            n128 = Format Into String(format string="%s %.1f %s", "Setting wavelength to" ("input 1"), w83, "nm ..." ("input 3")) -> (resulting string=w86:string, error out=w87:errorcluster)  [unwired: 2 in]
            n129 = call "Status Updated.vi"("error in (no error)"=w87, "Status"=w86) -> ("error out"=w82:errorcluster)  [unwired: 9 in]
            n130 = call-poly <vilib>:"Delacor_lib_QMH_Enqueue Message (poly).vi"("error in (no error)"=w82, "Message Data"=w92, "Message"="Set Wavelength", "Message Queue in"=w95) -> ("error out"=w89:errorcluster)  [unwired: 6 in, 1 out]
          }
          event User Event {
            # "Another Module called the \"Set Slit Width\" API Method."
            n131 = event-data() -> ("Slit Width (um)"=w97:dbl, "Wait Notifier"=w103:refnum<notifier>, "wait for reply"=w104:bool)  [unwired: 1 in]
            n132 = Bundle(cluster=T6 {"Slit Width (um)"=0.0, "Wait Notifier"=refnum, "wait for reply"=FALSE} ("Set Slit Width Argument"), "Slit Width (um)"=w97, "Wait Notifier"=w103, "wait for reply"=w104) -> (w106:T6)
            n133 = Format Into String(format string="%s %.1f %s", "Setting slit width to" ("input 1"), w97, "um ..." ("input 3")) -> (resulting string=w100:string, error out=w101:errorcluster)  [unwired: 2 in]
            n134 = call "Status Updated.vi"("error in (no error)"=w101, "Status"=w100) -> ("error out"=w96:errorcluster)  [unwired: 9 in]
            n135 = call-poly <vilib>:"Delacor_lib_QMH_Enqueue Message (poly).vi"("error in (no error)"=w96, "Message Data"=w106, "Message"="Set Slit Width", "Message Queue in"=w109) -> ("error out"=w105:errorcluster)  [unwired: 6 in, 1 out]
          }
          event User Event {
            # "Another Module called the \"Set Grating\" API Method."
            n136 = event-data() -> ("Grating ID"=w110:u32, "Wait Notifier"=w119:refnum<notifier>, "wait for reply"=w118:bool)  [unwired: 1 in]
            n137 = Bundle(cluster=T7 {"Grating ID"=0, "Wait Notifier"=refnum, "wait for reply"=FALSE} ("Set Grating Argument"), "Grating ID"=w110, "Wait Notifier"=w119, "wait for reply"=w118) -> (w120:T7)
            n138 = Format Into String(format string="%s %u %s", "Setting grating to ID" ("input 1"), w110, "..." ("input 3")) -> (resulting string=w115:string, error out=w116:errorcluster)  [unwired: 2 in]
            n139 = call "Status Updated.vi"("error in (no error)"=w116, "Status"=w115) -> ("error out"=w113:errorcluster)  [unwired: 9 in]
            n140 = call-poly <vilib>:"Delacor_lib_QMH_Enqueue Message (poly).vi"("error in (no error)"=w113, "Message Data"=w120, "Message"="Set Grating", "Message Queue in"=w123) -> ("error out"=w117:errorcluster)  [unwired: 6 in, 1 out]
          }
          event User Event {
            # "Another Module called the \"Get Module Data\" API Method."
            n141 = event-data() -> ("Wait Notifier"=w126:refnum<notifier>, "wait for reply"=w125:bool)  [unwired: 1 in]
            n142 = Bundle(cluster=T8 {"Wait Notifier"=refnum, "wait for reply"=FALSE} ("Get Module Data Argument"), "Wait Notifier"=w126, "wait for reply"=w125) -> (w127:T8)
            n143 = call-poly <vilib>:"Delacor_lib_QMH_Enqueue Message (poly).vi"("Message Data"=w127, "Message"="Get Module Data", "Message Queue in"=w130) -> ("error out"=w124:errorcluster)  [unwired: 7 in, 1 out]
          }
        }
        n144 = call-dynamic "Delacor_lib_QMH_Error Handler - Event Handling Loop.vi"("error in (no error)"=w32, "Message Queue in"=w26) -> ("dup error in"=w31:errorcluster)  [unwired: 8 in, 1 out]
      }
    }
    frame Error {
      # "Synchronize Caller Events.vi will inform Start Module.vi that the module has launched and will let the code calling Start Module.vi register for broadcasts and would permit the caller receive the broadcast that an error occurred at launch time."
      n145 = call-dynamic "Delacor_lib_QMH_Release Message Queue.vi"("error in (no error)"=w326, "Message Queue"=w324) -> ("error out"=w325:errorcluster)  [unwired: 9 in]
      n146 = call "Synchronize Caller Events.vi"("Singleton Module Admin in"=w327) -> ("error out"=w332:errorcluster)  [unwired: 9 in, 1 out]
      n147 = call "Module Name--constant.vi"() -> ("Module Name"=w330:string)  [unwired: 11 in]
      n148 = Format Into String(format string="An error occurred during initialization. %s is no longer running.", w330) -> (resulting string=w328:string)  [unwired: 2 in, 1 out]
      n149 = Merge Errors(w325, w332) -> (w333:errorcluster)
      n150 = call "Error Reported.vi"("Additional Information"=w328, "Error"=w333) -> ()  [unwired: 9 in, 1 out]
    }
  }
  n151 = Merge Errors(w14, w17) -> (w13:errorcluster)
  n152 = call "Close Module.vi"("error in (no error)"=w13, "Module Admin in"=w8) -> ("error out"=w15:errorcluster, "External Launch"=w1:bool, "Module Admin out"=w2:refnum<class "Delacor_lib_QMH_Module Admin.lvclass">)  [unwired: 7 in]
  n153 = Unregister For Events(event registration refnum=w7, error in=w15) -> (error out=w12:errorcluster)
  "error out" <- w12
  n154 = case "External Launch?" shown="True" w1 {
    tunnel: w12 -> [_ w334]
    frame False {
    }
    frame True {
      n155 = case shown="No Error" w334 {
        frame No Error {
          n156 = invoke class="VI" method="FP.Close"() -> ()  [unwired: 3 in, 3 out]
        }
        frame Error {
          n157 = invoke class="VI" method="FP.Open"("Activate"=TRUE ("Activate?")) -> ()  [unwired: 4 in, 5 out]
        }
      }
    }
  }
  n158 = local write "Module Admin"(w2) -> ()
